vi "util_SetFilterWheelPosition.vi"(8 "Filter Position":i8, 9 "Filter Transmission":dbl, 10 "Mode":enum16{"Set Position", "Set Transmission"}(ring)=enum."Set Transmission", 11 "Filter Wheel":enum16{"473nm", "532nm"}(ring)=enum."532nm") -> (3 "Success":bool)   [LabVIEW 2012]
uses:
  <vilib>/Utility/error.llb/DialogType.ctl
  <vilib>/Utility/error.llb/Error Cluster From Error Code.vi
  <vilib>/ErrorRing/Error Ring.xnode
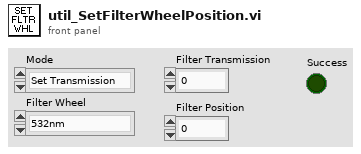
[diagram p1: front panel]
types:
  T1 = typedef "DialogType.ctl" = u16
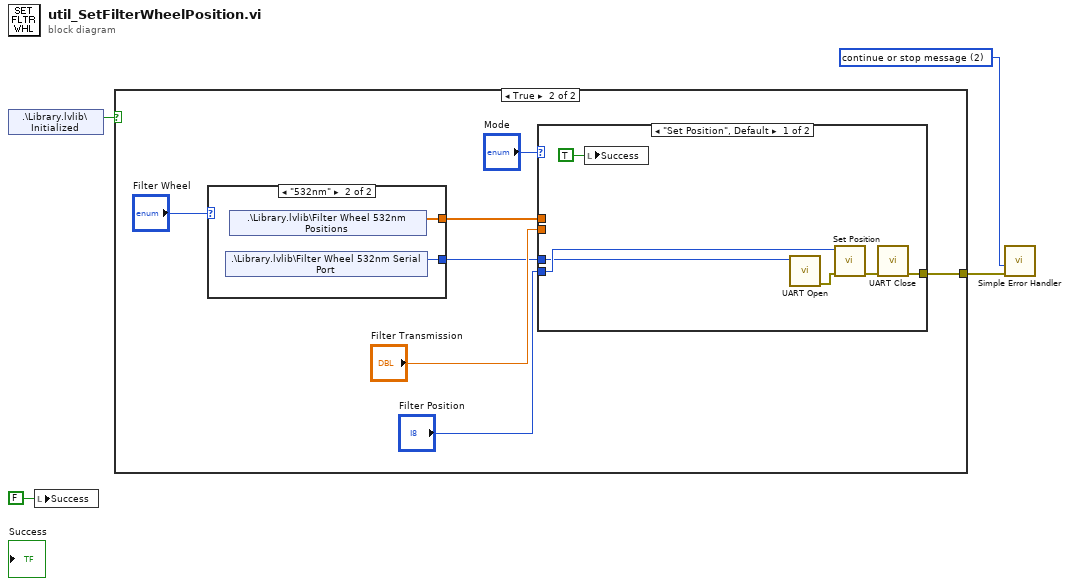
[diagram p0: block diagram]
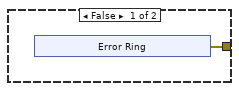
[diagram p2: hidden frame]
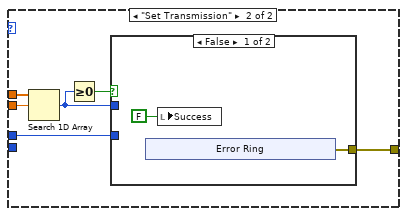
[diagram p3: hidden frame]
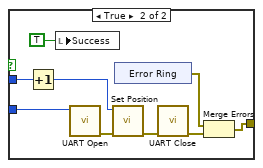
[diagram p4: hidden frame]
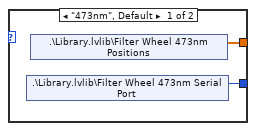
[diagram p5: hidden frame]
diagram:
  w1 = T1 2 items=["no dialog", "OK message", "continue or stop message", "OK message + warnings", "continue/stop + warnings"] ("type of dialog (OK msg:1)")
  n1 = shared-variable ".\\Library.lvlib\\Initialized"() -> (w3:bool)  [unwired: 1 in, 1 out]
  n2 = local write "Success"(FALSE ("Success")) -> ()
  n3 = case shown="True" w3 {
    tunnel: [w5 w11] -> w2
    frame False {
      n4 = xnode "Error Ring"() -> ("error out"=w5:errorcluster)
    }
    frame True {
      n5 = case shown="\"532nm\"" "Filter Wheel" {
        tunnel: [w48 w50] -> w12
        tunnel: [w47 w49] -> w15
        frame "473nm", Default {
          n6 = shared-variable ".\\Library.lvlib\\Filter Wheel 473nm Serial Port"() -> (w48:i8)  [unwired: 1 in, 1 out]
          n7 = shared-variable ".\\Library.lvlib\\Filter Wheel 473nm Positions"() -> (w47:dbl[])  [unwired: 1 in, 1 out]
        }
        frame "532nm" {
          n8 = shared-variable ".\\Library.lvlib\\Filter Wheel 532nm Serial Port"() -> (w50:i8)  [unwired: 1 in, 1 out]
          n9 = shared-variable ".\\Library.lvlib\\Filter Wheel 532nm Positions"() -> (w49:dbl[])  [unwired: 1 in, 1 out]
        }
      }
      n10 = case shown="\"Set Position\", Default" "Mode" {
        tunnel: w15 -> [_ w28]
        tunnel: "Filter Transmission" -> [_ w29]
        tunnel: "Filter Position" -> [w21 _]
        tunnel: w12 -> [w20 w27]
        tunnel: [w18 w24] -> w11
        frame "Set Position", Default {
          n11 = local write "Success"(TRUE ("Success")) -> ()
          n12 = call "UART Open.vi"("Serial Port"=w20) -> ("error out"=w23:errorcluster)  [unwired: 9 in, 1 out]
          n13 = call "Set Position.vi"("error in (no error)"=w23, "Position"=w21) -> ("error out"=w22:errorcluster)  [unwired: 9 in]
          n14 = call "UART Close.vi"("error in (no error)"=w22) -> ("error out"=w18:errorcluster)  [unwired: 10 in]
        }
        frame "Set Transmission" {
          n15 = Search 1D Array(1D array=w28, element=w29) -> (index of element=w26:i32)  [unwired: 1 in]
          n16 = Greater Or Equal To 0?(x=w26) -> (x >= 0?=w25:bool)
          n17 = case shown="False" w25 {
            tunnel: w27 -> [_ w43]
            tunnel: w26 -> [_ w40]
            tunnel: [w30 w37] -> w24
            frame False {
              n18 = xnode "Error Ring"() -> ("error out"=w30:errorcluster)
              n19 = local write "Success"(FALSE ("Success")) -> ()
            }
            frame True {
              n20 = Increment(x=w40) -> (x+1=w42:i32)
              n21 = local write "Success"(TRUE ("Success")) -> ()
              n22 = call "UART Open.vi"("Serial Port"=w43) -> ("error out"=w45:errorcluster)  [unwired: 9 in, 1 out]
              n23 = call "Set Position.vi"("error in (no error)"=w45, "Position"=w42) -> ("error out"=w44:errorcluster)  [unwired: 9 in]
              n24 = xnode "Error Ring"() -> ("error out"=w39:errorcluster)
              n25 = call "UART Close.vi"("error in (no error)"=w44) -> ("error out"=w38:errorcluster)  [unwired: 10 in]
              n26 = Merge Errors(w39, w38) -> (w37:errorcluster)
            }
          }
        }
      }
    }
  }
  n27 = call <vilib>:"Simple Error Handler.vi"("type of dialog (OK msg:1)"=w1, "error in (no error)"=w2) -> ()  [unwired: 3 in, 5 out]
